vi "Read Cache.vi"(11 "URI in":refnum<class "URI.lvclass">) -> (2 "Cache":string, 3 "URI out":refnum<class "URI.lvclass">)   [LabVIEW 2013, in "openURI.lvlib" / "URI.lvclass"]
uses:
  URI.lvclass
  URI.lvclass/URI.ctl
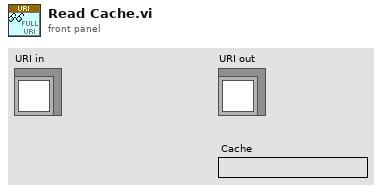
[diagram p1: front panel]
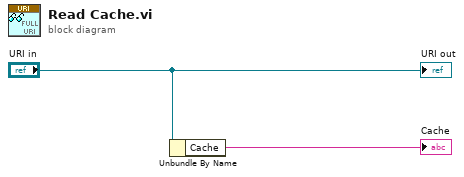
[diagram p0: block diagram]
diagram:
  n1 = Unbundle By Name("URI in") -> ("Cache"=→"Cache":string)
  "URI out" <- "URI in"
